vi "Queued Pedestrian Lights Second Loop.vi"() -> ()   [LabVIEW 2012]
doc: "Traffic Light VI with the use of Queues and LoadTrafficLightsQueue (with Exit) to Enqueue the Walk Element at the front of the Queue. Has control over both the Traffic Lights display and the Pedestrian Lights Display. Red is set as the initial State.\nNamed Second Loop as it uses second Loop to use an Event Structure to change the Waiting Indicator."
uses:
  Controls/Traffic Light Display.ctl
  Controls/Pedestrian Light Display.ctl
  Controls/Traffic Light States (with Walk and Exit State).ctl
panel:
  in  "Stop Button":bool
  out "Pedestrian Light Display":T1
  in  "Walk":bool
  out "Traffic Light Display":T2
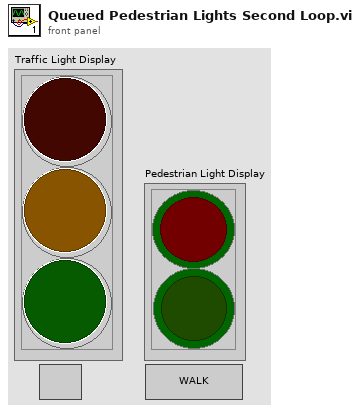
[diagram p1: front panel]
types:
  T1 = typedef "Pedestrian Light Display.ctl" = cluster{"Red":bool, "Green":bool}
  T2 = typedef "Traffic Light Display.ctl" = cluster{"RED":bool, "AMBER":bool, "GREEN":bool}
  T3 = typedef "Traffic Light States (with Walk and Exit State).ctl" = enum16{"Red", "RedAmber", "Green", "Amber", "Walk", "Exit"}
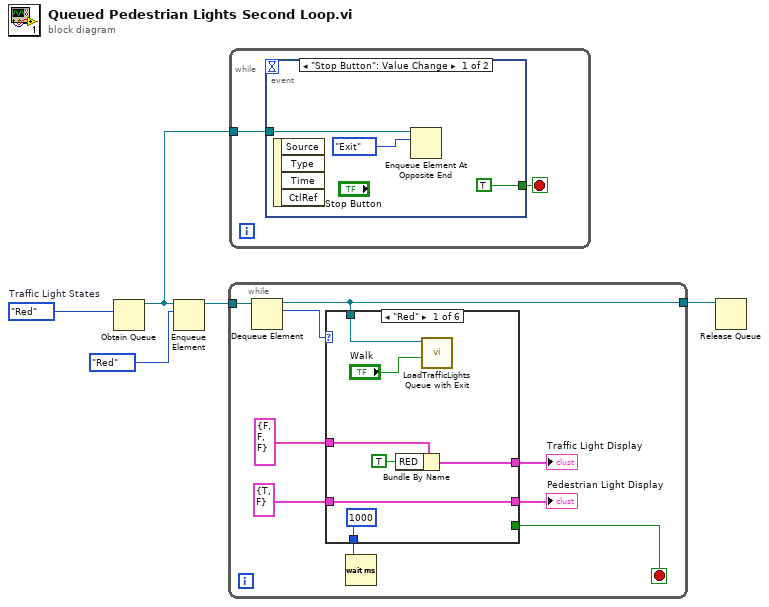
[diagram p0: block diagram]
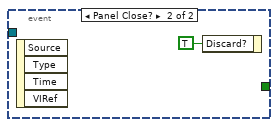
[diagram p2: hidden frame]
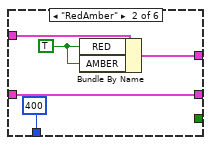
[diagram p3: hidden frame]
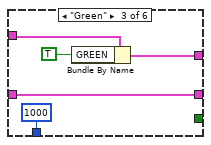
[diagram p4: hidden frame]
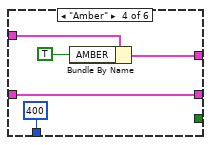
[diagram p5: hidden frame]
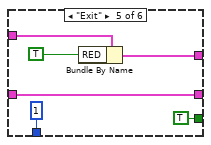
[diagram p6: hidden frame]
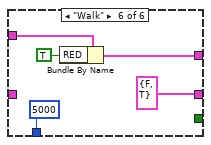
[diagram p7: hidden frame]
diagram:
  w2 = Traffic_Light_States_(with_Walk_and_Exit_State)."Red"  # Traffic Light States
  n1 = Obtain Queue(element data type=w2) -> (queue out=w4:refnum<queue>)  [unwired: 4 in, 2 out]
  n2 = Enqueue Element(queue=w4, element=Traffic_Light_States_(with_Walk_and_Exit_State)."Red" ("Traffic Light States")) -> (queue out=w5:refnum<queue>)  [unwired: 2 in, 2 out]
  n3 = while {
    tunnel: w5 -> [w9]
    tunnel: [w7] -> w3
    stop <- w6 stop-if-true
    n4 = Dequeue Element(queue=w9) -> (queue out=w7:refnum<queue>, element=w8:T3)  [unwired: 2 in, 2 out]
    n5 = case shown="\"Red\"" w8 {
      tunnel: T2 {"RED"=FALSE, "AMBER"=FALSE, "GREEN"=FALSE} ("Traffic Light Display") -> [w21 w26 w31 w36 w42 w46]
      tunnel: [w19 w25 w29 w34 w40 w44] -> w13
      tunnel: [1000 400 1000 400 1 5000] -> w12
      tunnel: T1 {"Red"=TRUE, "Green"=FALSE} ("Pedestrian Light Display") -> [w17 w23 w27 w32 w38 _]
      tunnel: [w17 w23 w27 w32 w38 T1 {"Red"=FALSE, "Green"=TRUE} ("Pedestrian Light Display")] -> w10
      tunnel: w7 -> [w16 _ _ _ _ _]
      tunnel: [_ _ _ _ TRUE _] -> w6
      frame "Red" {
        n6 = Bundle By Name(cluster=w21, "RED"=TRUE) -> (w19:T2)
        n7 = call "LoadTrafficLightsQueue with Exit.vi"("Queue Ref in"=w16, "Walk"="Walk") -> ()  [unwired: 9 in]
      }
      frame "RedAmber" {
        w22 = TRUE ("RED")
        n8 = Bundle By Name(cluster=w26, "RED"=w22, "AMBER"=w22) -> (w25:T2)
      }
      frame "Green" {
        n9 = Bundle By Name(cluster=w31, "GREEN"=TRUE ("RED")) -> (w29:T2)
      }
      frame "Amber" {
        n10 = Bundle By Name(cluster=w36, "AMBER"=TRUE ("RED")) -> (w34:T2)
      }
      frame "Exit" {
        n11 = Bundle By Name(cluster=w42, "RED"=TRUE) -> (w40:T2)
      }
      frame "Walk" {
        n12 = Bundle By Name(cluster=w46, "RED"=TRUE) -> (w44:T2)
      }
    }
    "Traffic Light Display" <- w13
    "Pedestrian Light Display" <- w10
    n13 = Wait (ms)(milliseconds to wait=w12) -> ()  [unwired: 1 out]
  }
  n14 = while {
    tunnel: w4 -> [w48]
    stop <- w49 stop-if-true
    n15 = event shown="[0] \"Stop Button\": Value Change" {
      selector: _ -> [_ _]
      dyn-events: _ -> [_ _]
      timeout: _ -> [_ _]
      tunnel: [TRUE _] -> w49
      tunnel: w48 -> [w51 _]
      event "Stop Button": Value Change {
        n16 = event-data() -> ()  [unwired: 1 in, 4 out]
        n17 = Enqueue Element At Opposite End(queue=w51, element=Traffic_Light_States_(with_Walk_and_Exit_State)."Exit" ("Traffic Light States")) -> ()  [unwired: 2 in, 3 out]
      }
      event Panel Close? {
        n18 = event-data() -> ()  [unwired: 1 in, 4 out]
        n19 = event-data("Discard?"=TRUE) -> ()  [unwired: 1 in, 1 out]
      }
    }
  }
  n20 = Release Queue(queue=w3) -> ()  [unwired: 2 in, 3 out]
